vi "FindAccelAngle.vi"(6 "Z":dbl, 7 "Y":dbl, 8 "X":dbl) -> (2 "Roll":dbl, 5 "Pitch":dbl)   [LabVIEW 2014]
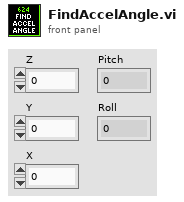
[diagram p1: front panel]
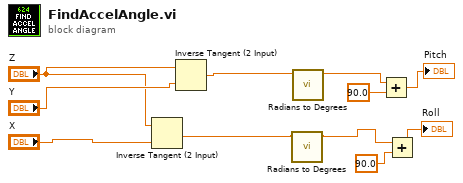
[diagram p0: block diagram]
diagram:
  n1 = Inverse Tangent (2 Input)(1:"X", 2:"Z") -> (0:w4:dbl)
  n2 = Inverse Tangent (2 Input)(1:"Y", 2:"Z") -> (0:w2:dbl)
  n3 = call "Radians to Degrees.vi"("Radians"=w4) -> ("Degrees"=w3:dbl)  [unwired: 10 in]
  n4 = call "Radians to Degrees.vi"("Radians"=w2) -> ("Degrees"=w1:dbl)  [unwired: 10 in]
  n5 = Add(x=w1, y=90.0) -> (x+y=→"Pitch":dbl)
  n6 = Add(x=w3, y=90.0) -> (x+y=→"Roll":dbl)
